vi "Intellifaucet-Start.vi"(7 "Semiphore":T1, 8 "Error In":errorcluster, 10 "mS wait":u32=200, 11 "VISA session":refnum<visa-resource-name>="MW100") -> (0 "Error Out":errorcluster, 3 "dup VISA session":refnum<visa-resource-name>)   [LabVIEW 2009]
uses:
  ChannelSettings.ctl
panel:
  out "Numeric":i32
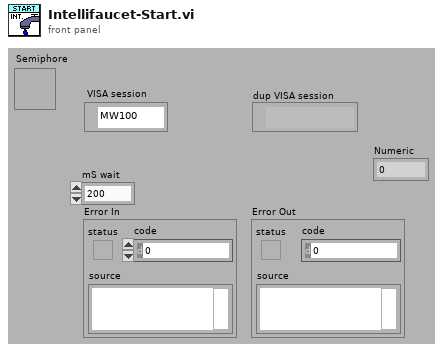
[diagram p1: front panel]
types:
  T1 = typedef "Semaphore RefNum" = refnum<k1>
  T2 = typedef "ChannelSettings.ctl" = u32
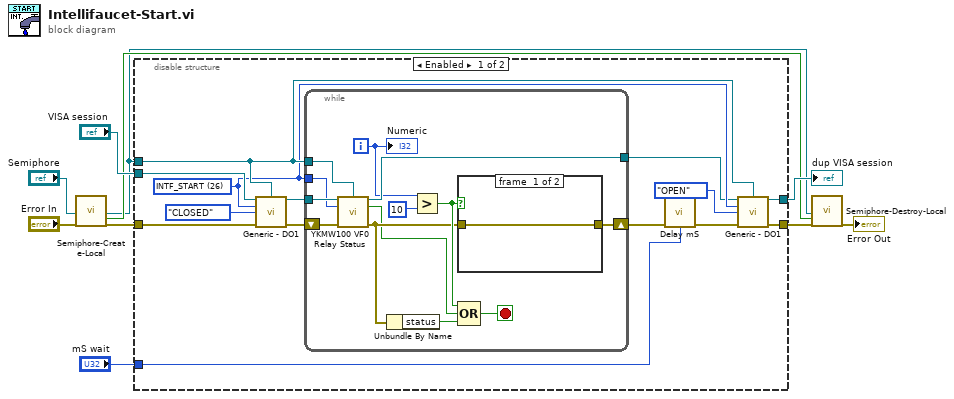
[diagram p0: block diagram]
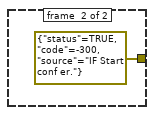
[diagram p2: hidden frame]
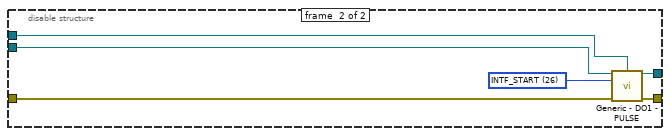
[diagram p3: hidden frame]
diagram:
  n1 = call "Semiphore-Create-Local.vi"("Semiphore"="Semiphore", "error in (no error)"="Error In") -> ("semaphore"=w1:T1, "Local?"=w4:bool, "error out"=w5:errorcluster)  [unwired: 15 in]
  n2 = disable-structure shown="Enabled" {
    disable-tunnel: "mS wait" -> [w24 _]
    disable-tunnel: "VISA session" -> [w20 w42]
    disable-tunnel: [w19 w43] -> w8
    disable-tunnel: w5 -> [w18 w45]
    disable-tunnel: [w17 w44] -> w3
    disable-tunnel: w1 -> [w14 w41]
    frame #0 {
      w13 = T2 26 items=["4-20_OUT", "Pres_HI1", "Pres_HI2", "Pres_LOW", "Pres_PIN", "HEATER_TOP", "HEATER_BOT", "T_Shell", "FLOWMETER", "WATT_SENSE", "WH_TICK", "Tc_1", "Tc_2", "Tc_3", "Tc_4", "Tc_5", "Tc_6", "Tc_down", "T_Shell_2", "T_Shell_3", "T_Shell_4", "RTD_IN", "RTD_OUT", "RTD_AMB", "INTF_TEMPFLO", "INTF_READY", "INTF_START", "INTF_STOP", "DRM_LOW", "DRM_HIGH", "PWR_MAIN", "VLV_DUMP", "VLV_OUT", "VLV_IN", "WATT_HOURS", "FLOW(SAMPLE)", "GALLONS", "FLOW(GPM)"] ("Channel_Enum")
      n3 = call "Generic - DO1.vi"("VISA session"=w20, "Semiphore"=w14, "Channel_Enum"=w13, "Relay Status (0:CLOSED)"=enum8{"CLOSED", "OPEN"}."CLOSED", "Error In"=w18) -> ("dup VISA session"=w16:refnum<visa-resource-name>, "error out"=w15:errorcluster)  [unwired: 9 in]
      n4 = while {
        tunnel: w16 -> [w37]
        tunnel: w14 -> [w36]
        tunnel: [w35] -> w11
        shift-right: [w27] -> w12
        shift-left: w15 -> [w33]
        tunnel: w13 -> [w34]
        i -> [w30]
        stop <- w31 stop-if-true
        n5 = call "YKMW100 VF0 Relay Status.vi"("VISA session"=w37, "Semiphore"=w36, "Channel_Enum"=w34, "error in (no error)"=w33) -> ("dup VISA session"=w35:refnum<visa-resource-name>, "Output On"=w25:bool, "error out"=w26:errorcluster)  [unwired: 8 in, 1 out]
        n6 = Unbundle By Name(w26) -> ("status"=w32:bool)
        n7 = Greater?(x=w30, y=10) -> (0:w28:bool)
        n8 = case shown="True" w28 {
          tunnel: [w38 errorcluster {"status"=TRUE, "code"=-300, "source"="IF Start conf er."} ("error out")] -> w27
          tunnel: w26 -> [w38 _]
          frame #0 {
          }
          frame #1 {
          }
        }
        n9 = Compound Arithmetic op=OR(w28, w25, w32) -> (w31:bool)
        "Numeric" <- w30
      }
      n10 = call "Delay mS.vi"("Error In"=w12, "milliseconds to wait"=w24) -> ("Error Out"=w23:errorcluster)  [unwired: 13 in]
      n11 = call "Generic - DO1.vi"("VISA session"=w11, "Semiphore"=w14, "Channel_Enum"=w13, "Relay Status (0:CLOSED)"=enum8{"CLOSED", "OPEN"}."OPEN", "Error In"=w23) -> ("dup VISA session"=w19:refnum<visa-resource-name>, "error out"=w17:errorcluster)  [unwired: 9 in]
    }
    frame #1 {
      w40 = T2 26 items=["4-20_OUT", "Pres_HI1", "Pres_HI2", "Pres_LOW", "Pres_PIN", "HEATER_TOP", "HEATER_BOT", "T_Shell", "FLOWMETER", "WATT_SENSE", "WH_TICK", "Tc_1", "Tc_2", "Tc_3", "Tc_4", "Tc_5", "Tc_6", "Tc_down", "T_Shell_2", "T_Shell_3", "T_Shell_4", "RTD_IN", "RTD_OUT", "RTD_AMB", "INTF_TEMPFLO", "INTF_READY", "INTF_START", "INTF_STOP", "DRM_LOW", "DRM_HIGH", "PWR_MAIN", "VLV_DUMP", "VLV_OUT", "VLV_IN", "WATT_HOURS", "FLOW(SAMPLE)", "GALLONS", "FLOW(GPM)"] ("Channel_Enum")
      n12 = call "Generic - DO1 - PULSE.vi"("VISA session"=w42, "Semiphore"=w41, "Channel_Enum"=w40, "Error In"=w45) -> ("dup VISA session"=w43:refnum<visa-resource-name>, "error out"=w44:errorcluster)  [unwired: 10 in]
    }
  }
  "dup VISA session" <- w8
  n13 = call "Semiphore-Destroy-Local.vi"("Semiphore"=w1, "Local?"=w4, "error in (no error)"=w3) -> ("error out"=→"Error Out":errorcluster)  [unwired: 16 in]
